vi "Done.vi"(8 "error in (no error)":errorcluster, 11 "Asynchronous Application Log in":refnum<class "Asynchronous Application Log.lvclass">) -> (0 "error out":errorcluster, 3 "Asynchronous Application Log out":refnum<class "Asynchronous Application Log.lvclass">)   [LabVIEW 2016, in "Stream Log.lvlib" / "Asynchronous Application Log.lvclass"]
doc: "--\nCopyright © 2017 Composed SystemsI All rights reserved.\n\nAuthor: Jon McBee <jon.mcbee@composed.io>\n\nThis library is provided \"AS IS\" ,WITHOUT WARRANTIES OR\nCONDITIONS OF ANY KIND, either express or implied.\n\nComposed Systems -- composed.io\n\nStream 0.0.1.1\nJon McBee - Composed Systems\nCopyright (c) 2017, Composed Systems"
uses:
  <userlib>/Composed Systems/Stream/Log/Asynchronous Application Log/Asynchronous Application Log.lvclass
  <userlib>/Composed Systems/Stream/Log/Asynchronous Application Log/Message.ctl
  <userlib>/Composed Systems/Stream/Log/Asynchronous Application Log/Entry Type.ctl
  <userlib>/Composed Systems/Stream/Log/Log Sink/Log Sink.lvclass
  <userlib>/Composed Systems/Stream/Log/Asynchronous Application Log/Asynchronous Application Log.lvclass/Asynchronous Application Log.ctl
  <userlib>/Composed Systems/Stream/Log/Application Log/Application Log.lvclass
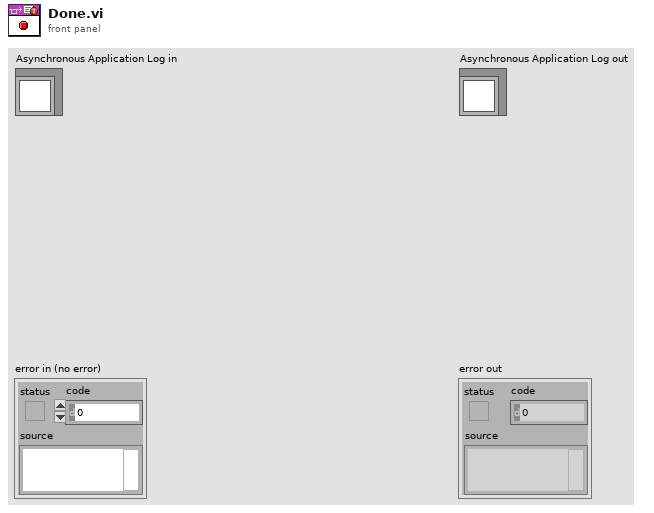
[diagram p1: front panel]
types:
  T1 = typedef "Stream Log.lvlib/Asynchronous Application Log.lvclass/Message.ctl" = cluster{"Entry Type":T2, "String":string, "Sinks":refnum<data-value>[], "Parallel Sinks?":bool}
  T2 = typedef "Stream Log.lvlib/Asynchronous Application Log.lvclass/Entry Type.ctl" = enum16{"Kill Worker", "Log Entry"}
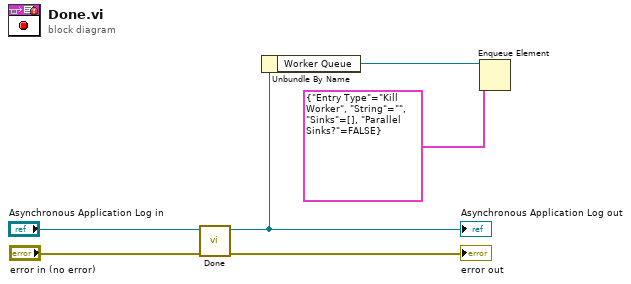
[diagram p0: block diagram]
diagram:
  n1 = call-parent "Done.vi"("error in (no error)"="error in (no error)", "Application Log in"="Asynchronous Application Log in") -> ("error out"=→"error out":errorcluster, "Application Log out"=w3:refnum<class "Asynchronous Application Log.lvclass">)  [unwired: 8 in]
  "Asynchronous Application Log out" <- w3
  n2 = Unbundle By Name(w3) -> ("Worker Queue"=w2:refnum<queue>)
  n3 = Enqueue Element(queue=w2, element=T1 {"Entry Type"=enum."Kill Worker", "String"="", "Sinks"=[], "Parallel Sinks?"=FALSE}) -> ()  [unwired: 2 in, 3 out]
